vi "Event to CSV String v2.vi"(8 "error in (no error)":errorcluster, 11 "Event":T1) -> (0 "error out":errorcluster, 2 "String":string)   [LabVIEW 2019, in "Logger.lvlib" / "Logger.lvclass"]
uses:
  Logger.lvclass
  Sensors/Detector/Event.ctl
  Sensors/Detector/Muon Detector.lvclass
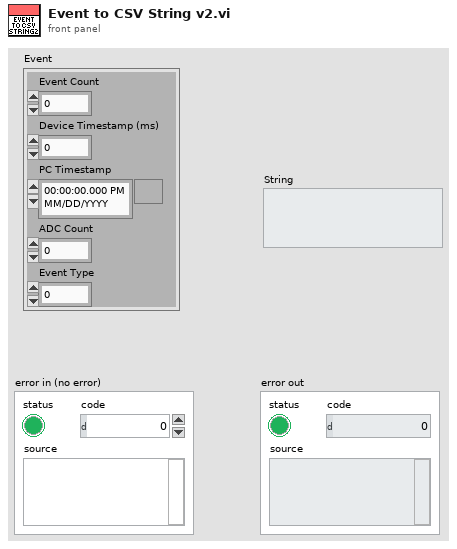
[diagram p1: front panel]
types:
  T1 = typedef "Muon Detector.lvclass/Event.ctl" = cluster{"Event Count":i32, "Device Timestamp (ms)":i32, "PC Timestamp":timestamp, "ADC Count":i32, "Event Type":u8}
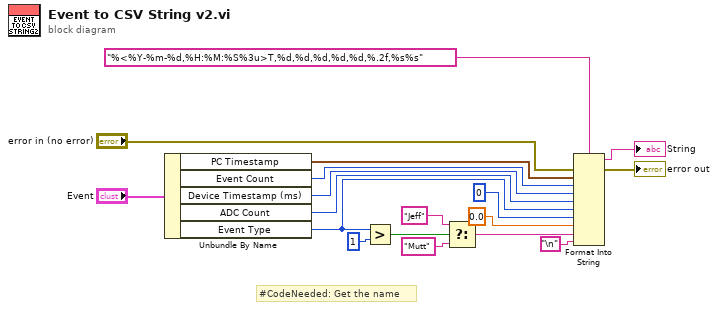
[diagram p0: block diagram]
diagram:
  # "#CodeNeeded: Get the name"
  n1 = Unbundle By Name("Event") -> ("PC Timestamp"=w1:timestamp, "Event Count"=w3:i32, "Device Timestamp (ms)"=w4:i32, "ADC Count"=w5:i32, "Event Type"=w7:u8)
  n2 = Greater?(x=w7, y=u8 1) -> (0:w9:bool)
  n3 = Select(t="Jeff", s=w9, f="Mutt") -> (s? t:f=w10:string)
  n4 = Format Into String(format string="%<%Y-%m-%d,%H:%M:%S%3u>T,%d,%d,%d,%d,%d,%.2f,%s%s", error in="error in (no error)", w1, w3, w4, w5, w7, 0 ("input 6"), 0.0, w10, "\n") -> (resulting string=→"String":string, error out=→"error out":errorcluster)  [unwired: 1 in]
